vi "CluseterTest.vi"() -> ()   [LabVIEW 2018]
panel:
  out "불리언 4":bool
  out "불리언 3":bool
  out "숫자형":i32
  out "문자열":string
  out "출력 클러스터":cluster{string, i32, bool, "불리언 2":bool}
  in  "불리언 2":bool
  out "연결된 문자열":string
  in  "배열":string[][](array[string])
  in  "정지":bool
  out "x .implies. y?":bool
  in  "불리언":bool
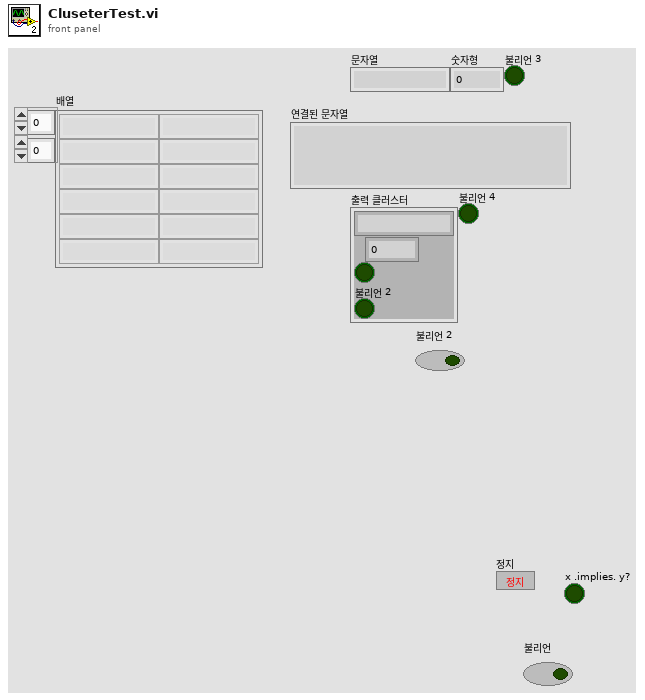
[diagram p1: front panel]
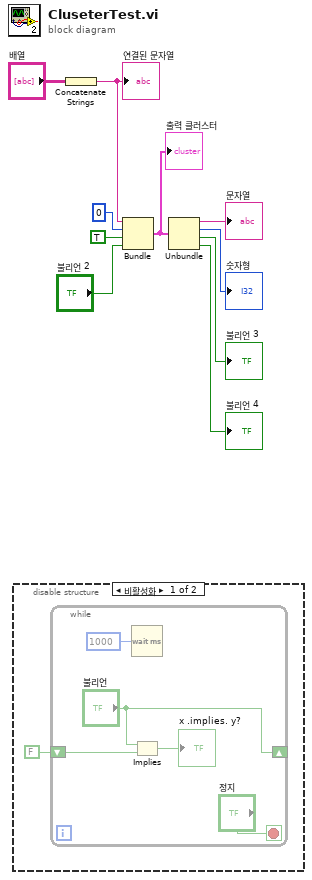
[diagram p0: block diagram]
diagram:
  n1 = disable-structure shown="비활성화" {
    frame Disabled {
      n2 = while {
        shift-right: ["불리언"] -> _
        shift-left: FALSE ("불리언") -> [w15]
        stop <- "정지" stop-if-true
        n3 = Wait (ms)(milliseconds to wait=u32 1000 ("대기 시간 (ms)")) -> ()  [unwired: 1 out]
        n4 = Implies(1:w15, 2:"불리언") -> (0:→"x .implies. y?":bool)
      }
    }
    frame Enabled {
    }
  }
  n5 = Concatenate Strings("배열") -> (w9:string)
  "연결된 문자열" <- w9
  n6 = Bundle(w9, 0, TRUE, "불리언 2"="불리언 2") -> (w5:cluster{string, i32, bool, "불리언 2":bool})  [unwired: 1 in]
  "출력 클러스터" <- w5
  n7 = Unbundle(w5) -> (→"문자열":string, →"숫자형":i32, →"불리언 3":bool, "불리언 2"=→"불리언 4":bool)
